vi "measure_valve_position.vi"(6 "error in":errorcluster) -> (0 "status":bool=TRUE, 3 "data":dbl[](array[numeric]), 4 "error out":errorcluster={"status"=TRUE, "code"=10023, "source"="ULx Create Channel (AI-Voltage-Basic).vi:5780001<ERR>\nMeasurements: Channel not specified."})   [LabVIEW 2019]
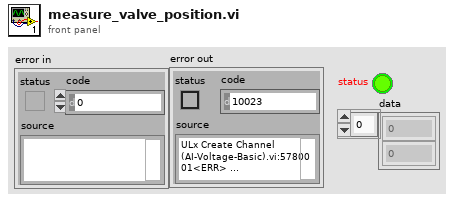
[diagram p1: front panel]
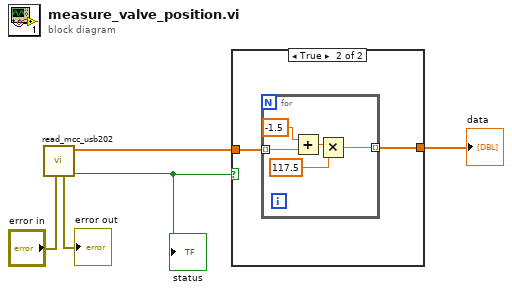
[diagram p0: block diagram]
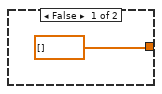
[diagram p2: hidden frame]
diagram:
  n1 = call "read_mcc_usb202.vi"("error in"="error in") -> ("status"=w3:bool, "data"=w1:dbl[], "error out"=→"error out":errorcluster)  [unwired: 8 in]
  "status" <- w3
  n2 = case shown="True" w3 {
    tunnel: [dbl[] [] ("data") w7] -> w2
    tunnel: w1 -> [_ w8]
    frame False {
    }
    frame True {
      n3 = for {
        tunnel: w8 -> [w13] mode=indexing
        tunnel: [w9] -> w7 mode=indexing
        n4 = Add(x=-1.5, y=w13) -> (x+y=w11:dbl)
        n5 = Multiply(x=w11, y=117.5) -> (x*y=w9:dbl)
      }
    }
  }
  "data" <- w2
